vi "FTW-Publisher-Construct.vi"(5 "Instance Inbox Address":string, 7 "Linger":i32=200 format="%d msec", 11 "error in":errorcluster) -> (4 "FTW Publisher":refnum<data-value>, 6 "Resolved Inbox Address":string, 15 "error out":errorcluster)   [LabVIEW 2015]
doc: "Performs a \"cold call\" to connect to a running Actor Instance at the given Instance Inbox Address. Normally, this method is wrapped by a \"Construct\" method in each specific Actor Connector subclass."
uses:
  core/FTW-Publisher-Core-Type.ctl
panel:
  # "Inputs"
  # "Outputs"
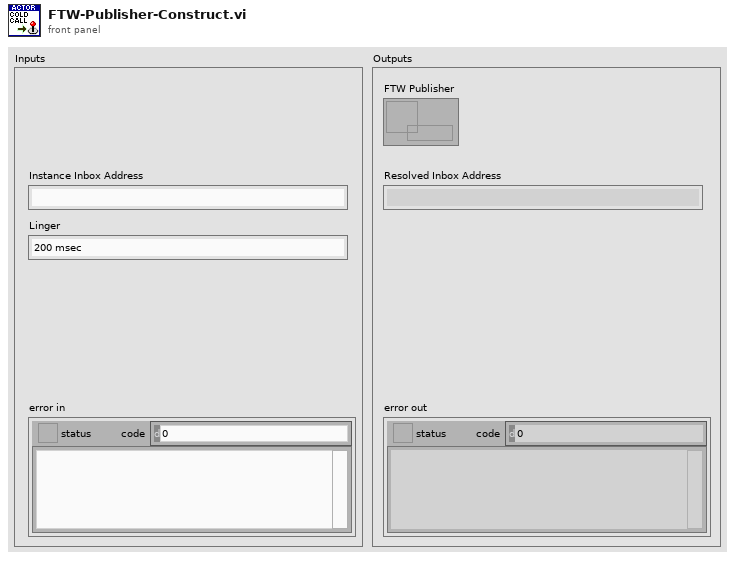
[diagram p1: front panel]
types:
  T1 = typedef "FTW-Publisher-Core-Type.ctl" = cluster{"Socket":i64}
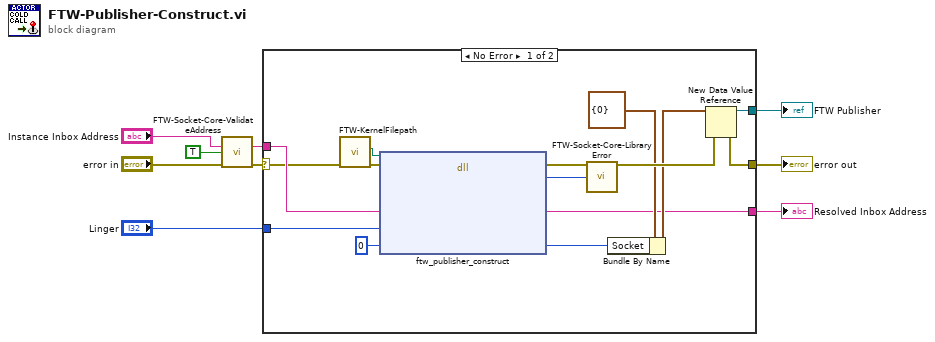
[diagram p0: block diagram]
diagram:
  n1 = call "FTW-Socket-Core-ValidateAddress.vi"("Address"="Instance Inbox Address", "Allow wildcard replacement?"=TRUE, "error in"="error in") -> ("Sanitized Address"=w4:string, "error out"=w5:errorcluster)  [unwired: 10 in, 1 out]
  n2 = case shown="No Error" w5 {
    selector: w5 -> [w12 w25]
    tunnel: [w22 w25] -> w9
    tunnel: w4 -> [w19 _]
    tunnel: [w21 _] -> w8
    tunnel: "Linger" -> [w16 _]
    tunnel: [w13 _] -> w1
    frame No Error {
      n3 = call "FTW-KernelFilepath.vi"("error in"=w12) -> ("error out"=w11:errorcluster, "Library Filepath"=w10:path)  [unwired: 8 in, 1 out]
      n4 = dll-call lib="?" fn="ftw_publisher_construct"(path in=w10, error in=w11, "Local Address"=w19, "Linger (msec)"=w16, "Socket Handle"=i64 0) -> (error out=w20:errorcluster, "Return Value"=w17:i64, "Local Address"=w13:string, "Socket Handle"=w14:i64)  [unwired: 4 in, 1 out]
      n5 = call "FTW-Socket-Core-LibraryError.vi"("error in"=w20, "Return Value"=w17) -> ("error out"=w24:errorcluster)  [unwired: 13 in]
      n6 = Bundle By Name(cluster=T1 {"Socket"=0} ("FTW Synchronous Server"), "Socket"=w14) -> (w15:T1)
      n7 = New Data Value Reference(data value=w15, error in=w24) -> (data value reference=w21:refnum<data-value>, error out=w22:errorcluster)
    }
    frame Error {
    }
  }
  "error out" <- w9
  "FTW Publisher" <- w8
  "Resolved Inbox Address" <- w1
